vi "LoadStratagems.vi"(8 "error in":errorcluster) -> (0 "error out":errorcluster, 2 "Array":string[](array[string]), 3 "Array 2":string[](array[string]))   [LabVIEW 2024]
uses:
  Controls/StratagemRing.ctl
panel:
  in  "Ring":u16(ring) items=[" 1 CP", " 1 CP", " 2 CP"]
  in  "Stratagems":T1 {"Cost" items=[" 1 CP", " 1 CP", " 2 CP"]; "Name" items=["Command Reroll", " Smoke", " Fire and Fade"]}
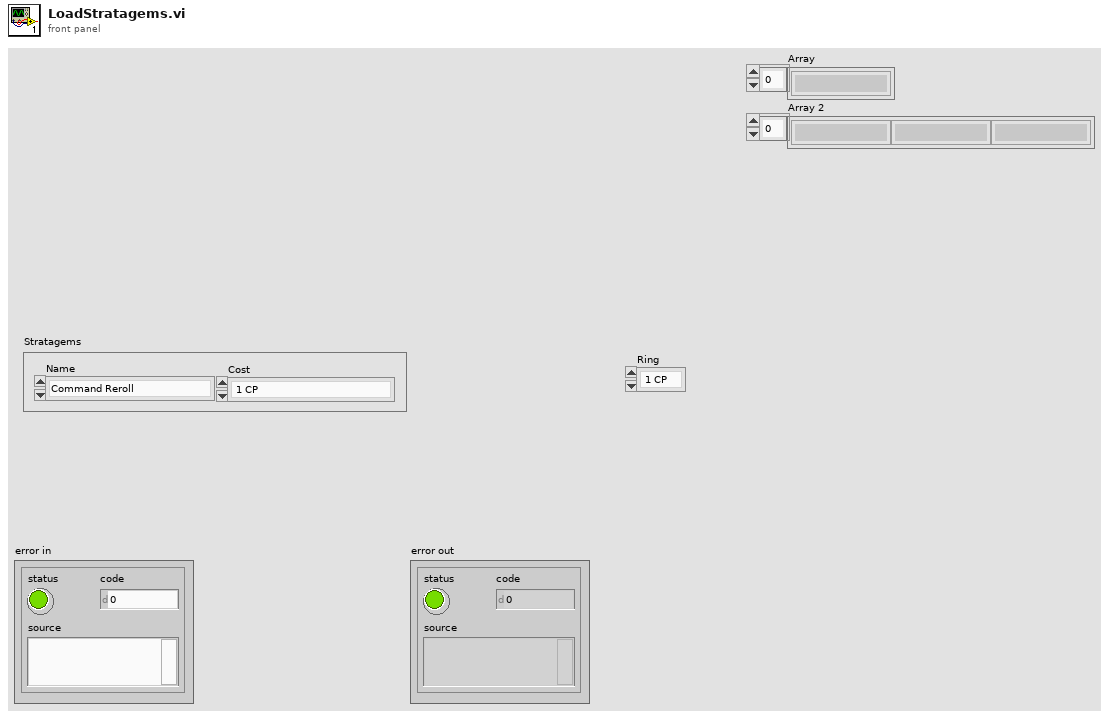
[diagram p1: front panel]
types:
  T1 = typedef "StratagemRing.ctl" = cluster{"Name":u16, "Cost":u16}
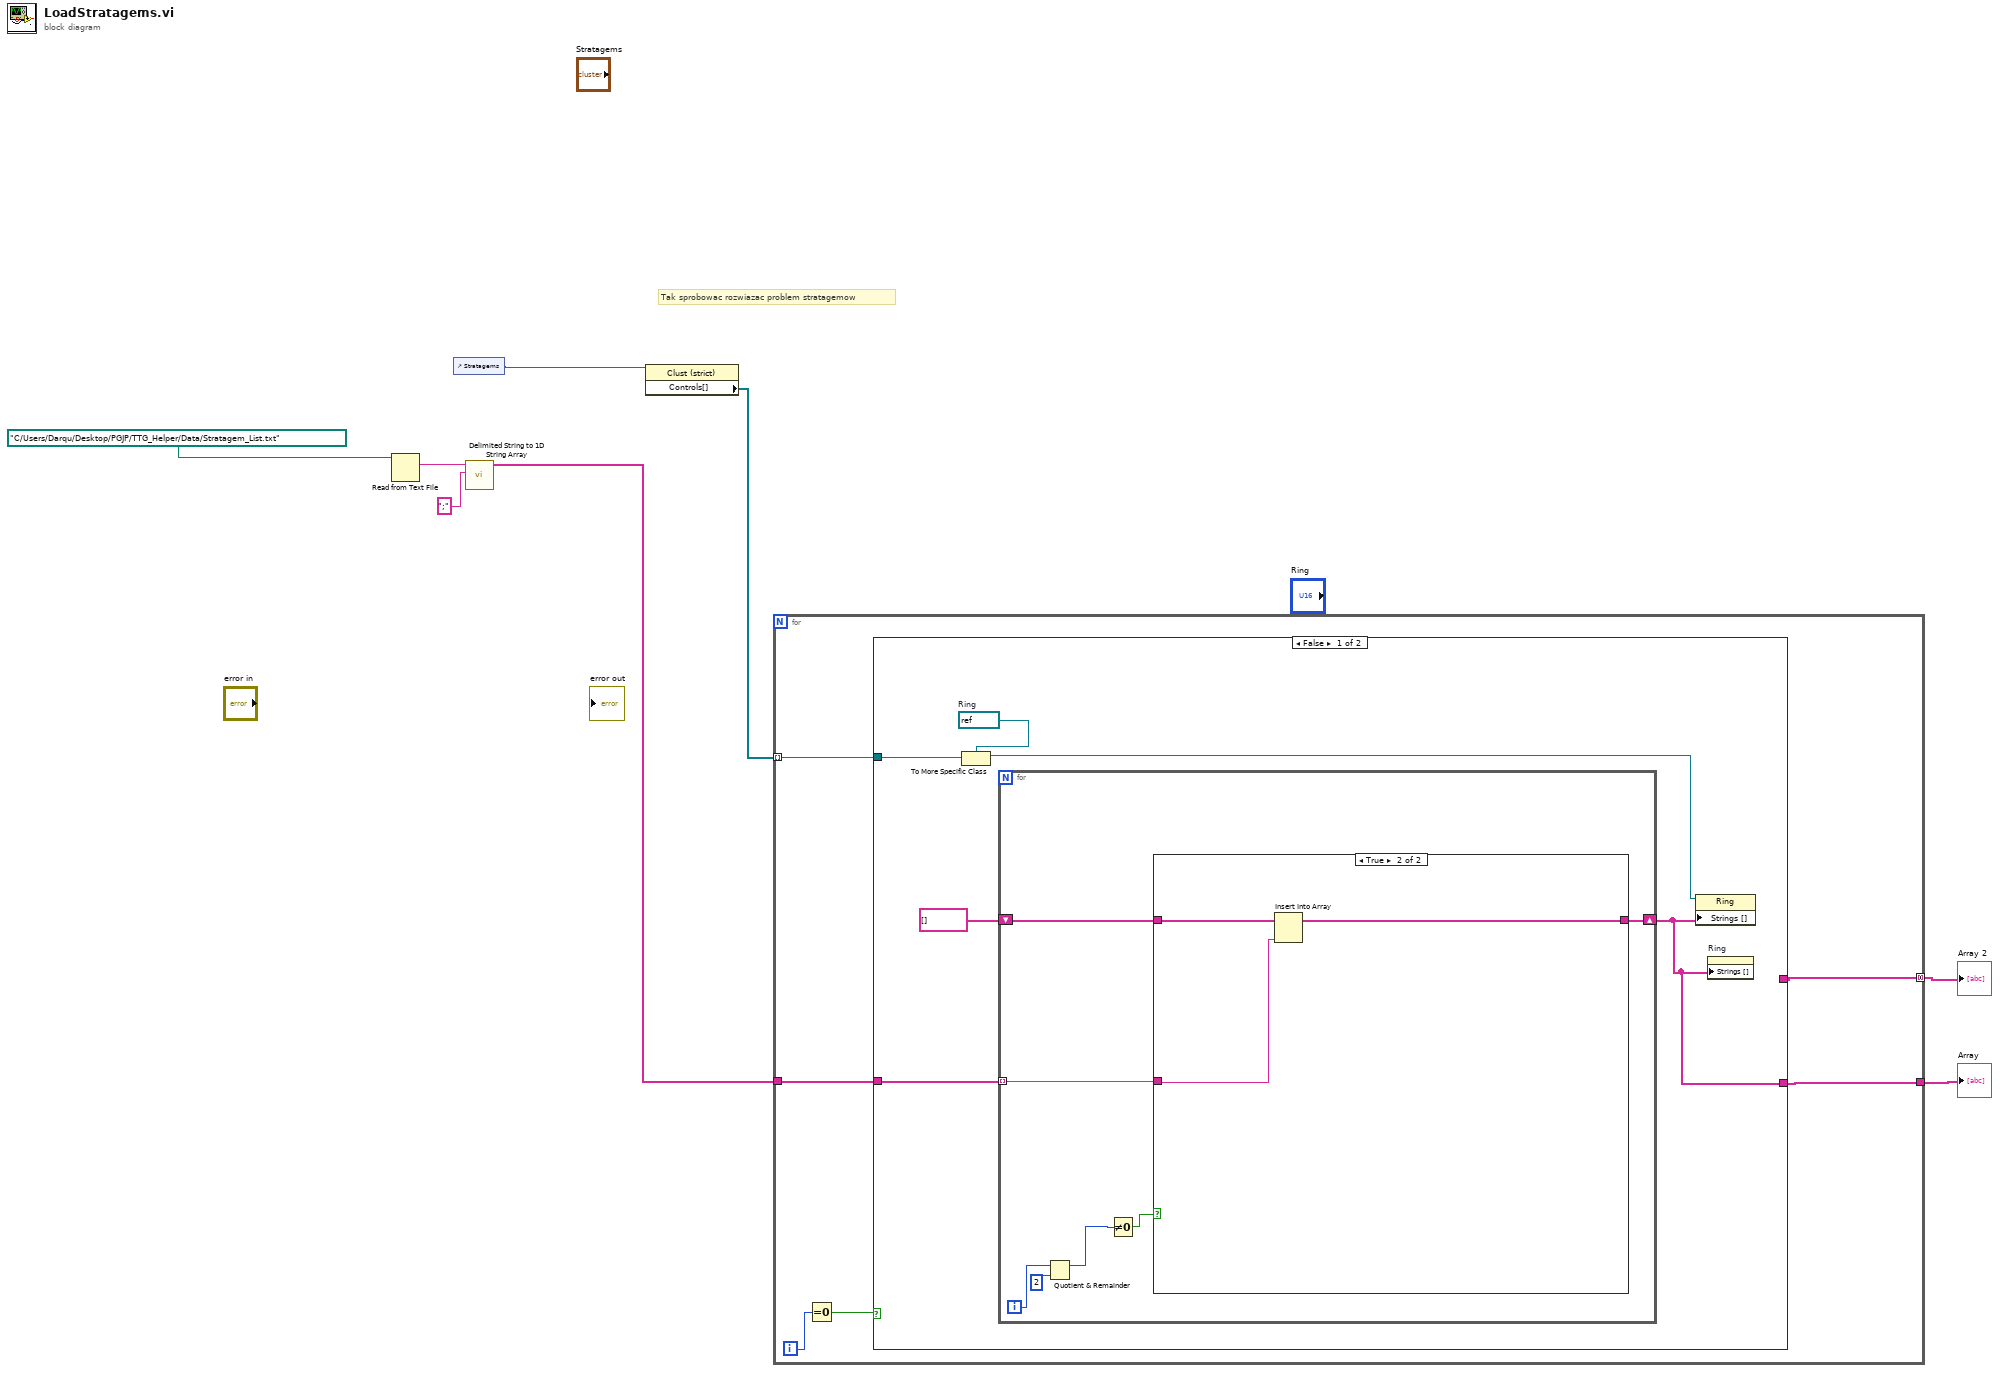
[diagram p0: block diagram]
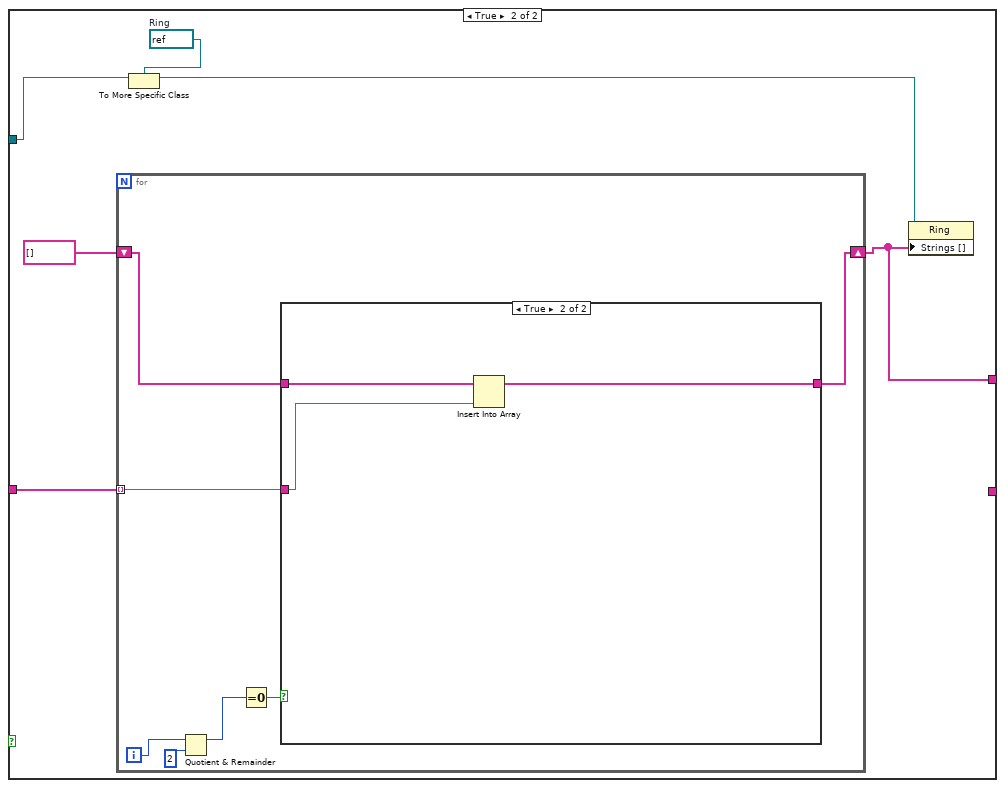
[diagram p3: hidden frame]
diagram:
  # "Tak sprobowac rozwiazac problem stratagemow"
  n1 = Read from Text File(file (use dialog)=path "C:/Users/Darqu/Desktop/PGJP/TTG_Helper/Data/Stratagem_List.txt") -> (text=w4:string)  [unwired: 3 in, 3 out]
  n2 = control-ref of="Stratagems"() -> (w7:refnum<vi>)
  n3 = call <vilib>:"Delimited String to 1D String Array.vi"("delimiter"=";", "delimited string"=w4) -> ("string array"=w6:string[])  [unwired: 9 in]
  n4 = property class="Clust (strict)"(reference=w7) -> ("Controls[]"=w8:refnum<vi>[])  [unwired: 1 in, 2 out]
  n5 = for {
    tunnel: w8 -> [w12] mode=indexing
    tunnel: w6 -> [w11]
    tunnel: [w10] -> w2
    tunnel: [w9] -> w1 mode=concatenating
    i -> [w14]
    n6 = Equal To 0?(x=w14) -> (x = 0?=w13:bool)
    n7 = case shown="False" w13 {
      tunnel: w12 -> [w19 w34]
      tunnel: w11 -> [w17 w37]
      tunnel: [w15 _] -> w10
      tunnel: [_ w32] -> w9
      frame False {
        w20 = refnum<vi> refnum  # Ring
        n8 = To More Specific Class(target class=w20, reference=w19) -> (specific class reference=w16:refnum<vi>)  [unwired: 1 in, 1 out]
        n9 = for {
          shift-right: [w21] -> w15
          shift-left: string[] [] -> [w22]
          tunnel: w17 -> [w27] mode=indexing
          i -> [w25]
          n10 = Quotient & Remainder(x=w25, y=2) -> (x-y*floor(x/y)=w24:i32)  [unwired: 1 out]
          n11 = Not Equal To 0?(x=w24) -> (x != 0?=w23:bool)
          n12 = case shown="True" w23 {
            tunnel: w27 -> [_ w29]
            tunnel: w22 -> [w28 w31]
            tunnel: [w28 w30] -> w21
            frame False {
            }
            frame True {
              n13 = Insert Into Array(array=w31, new element=w29) -> (w30:string[])  [unwired: 1 in]
            }
          }
        }
        n14 = property class="Ring"(reference=w16, "Strings []"=w15) -> ()  [unwired: 1 in, 2 out]
        n15 = property on="Ring" class="Ring (strict)"("Strings []"=w15) -> ()  [unwired: 2 in, 2 out]
      }
      frame True {
        w35 = refnum<vi> refnum  # Ring
        n16 = for {
          tunnel: w37 -> [w39] mode=indexing
          shift-right: [w38] -> w32
          shift-left: string[] [] -> [w40]
          i -> [w42]
          n17 = Quotient & Remainder(x=w42, y=2) -> (x-y*floor(x/y)=w44:i32)  [unwired: 1 out]
          n18 = Equal To 0?(x=w44) -> (x = 0?=w41:bool)
          n19 = case shown="True" w41 {
            tunnel: w40 -> [w45 w48]
            tunnel: w39 -> [_ w47]
            tunnel: [w45 w46] -> w38
            frame False {
            }
            frame True {
              n20 = Insert Into Array(array=w48, new element=w47) -> (w46:string[])  [unwired: 1 in]
            }
          }
        }
        n21 = To More Specific Class(target class=w35, reference=w34) -> (specific class reference=w36:refnum<vi>)  [unwired: 1 in, 1 out]
        n22 = property class="Ring"(reference=w36, "Strings []"=w32) -> ()  [unwired: 1 in, 2 out]
      }
    }
  }
  "Array" <- w2
  "Array 2" <- w1
